vi "Test1.vi"   [LabVIEW 2020]
uses:
  Fixture Enum.ctl
  Projects/Sensor Dispense.lvclass
  Fixture.lvclass
  Controller/Controller.lvclass
types:
  T1 = typedef "Fixture.lvclass/Fixture Enum.ctl" = enum16{"Assembly Tray", "Syringe Space", "Component", "Pick Up Tool", "Current Position"}
  T2 = typedef "Controller.lvclass/Controllers.ctl" = cluster{"I-O.lvclass":refnum<class "I-O.lvclass">, "Dispenser.lvclass":refnum<class "Dispenser.lvclass">, "Gantry":refnum<k24>}
  T3 = typedef "Fixture.lvclass/Workspace.ctl" = cluster{"XYZTheta":dbl[], "Workspace Valve":i32, "Workspace Sensor":i32}
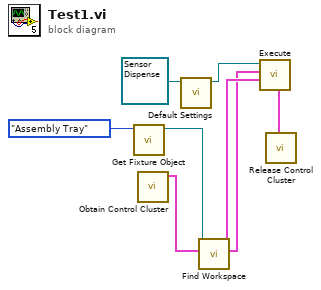
[diagram p0: block diagram]
diagram:
  n1 = call "Get Fixture Object.vi"("Fixture"=Fixture_Enum."Assembly Tray") -> ("Workspace.lvclass"=w1:refnum<class "Fixture.lvclass">)  [unwired: 8 in, 2 out]
  n2 = call "Obtain Control Cluster.vi"() -> ("Control Out"=w4:T2)  [unwired: 11 in]
  n3 = call-dynamic "Default Settings.vi"("Sensor Dispense in"=refnum<class "Sensor Dispense.lvclass"> refnum ("Sensor Dispense.lvclass")) -> ("Sensor Dispense out"=w5:refnum<class "Sensor Dispense.lvclass">)  [unwired: 9 in, 1 out]
  n4 = call-dynamic "Find Workspace.vi"("Control In"=w4, "Workspace In"=w1) -> ("Workspace Out"=w3:T3, "Control Out"=w2:T2)  [unwired: 6 in, 2 out]
  n5 = call-dynamic "Execute.vi"("Workspace"=w3, "Control In"=w2, "Dispense in"=w5) -> ("Control Out"=w8:T2)  [unwired: 6 in, 2 out]
  n6 = call "Release Control Cluster.vi"("output cluster"=w8) -> ()  [unwired: 11 in]
